vi "AuMT8852B Transmitter Test.vi"(7 "Settings":T1={"Pattern"=enum."10101010", "Hop type"=enum."Fixed", "TX/RX channel"=0, "Packet type"=enum."DH1", "Data length"=27, "Number of packets"=10}, 8 "error in (no error)":errorcluster, 11 "VISA session":refnum<visa-resource-name>) -> (0 "error out":errorcluster, 2 "error code":i32, 3 "VISA session out":refnum<visa-resource-name>)   [LabVIEW 2017]
doc: "Anritsu MT8852B Bluetooth Tester\n\nPerforms a single transmitter test control sequence. EUT must be in Test Mode before using this VI. Use Put EUT In Test Mode.vi.\n\nINPUTS\n Settings - parameters of the transmit test."
panel:
  # "Usage Notes: EUT must be in Test Mode before using this VI. Use Put EUT In Test Mode.vi."
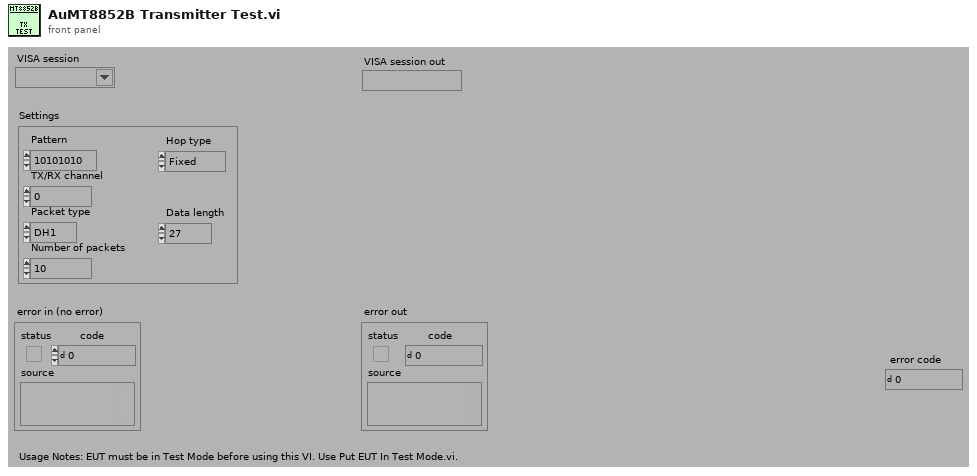
[diagram p1: front panel]
types:
  T1 = cluster{"Pattern":enum16{"10101010", "11110000", "PRBS-9"}, "Hop type":enum16{"Fixed", "Standard"}, "TX/RX channel":i32, "Packet type":enum16{"DH5", "DH3", "DH1"}, "Data length":i32, "Number of packets":i32}
  T2 = enum16{"Simulate", "Range check", "Cache", "Query instrument status"}
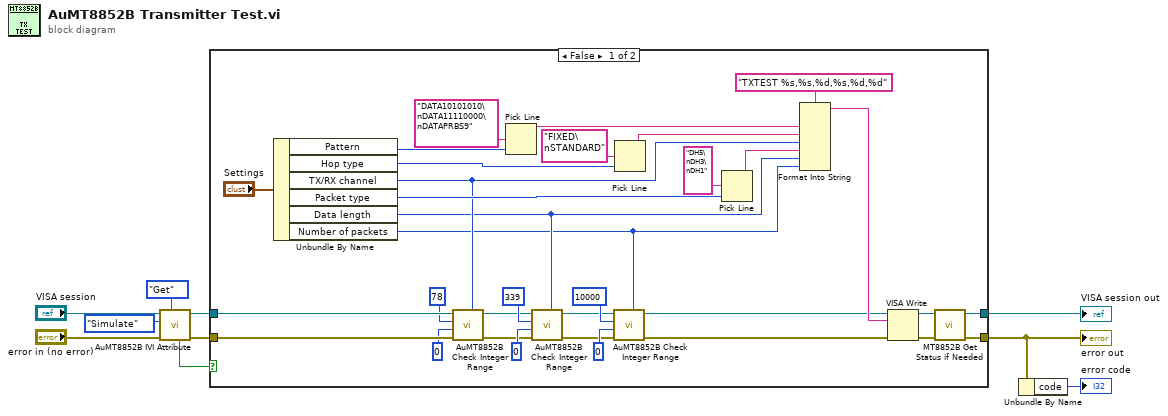
[diagram p0: block diagram]
diagram:
  n1 = call <instrlib>:"AuMT8852B IVI Attribute.vi"("Set/Get (Set)"=enum16{"Set", "Get"}."Get", "error in (no error)"="error in (no error)", "Flag (Simulate)"=T2."Simulate", "VISA session"="VISA session") -> ("error out"=w8:errorcluster, "VISA session out"=w9:refnum<visa-resource-name>, "Value out"=w3:bool)  [unwired: 5 in]
  n2 = case shown="False" w3 {
    tunnel: [w43 w45] -> w10
    tunnel: [w42 w44] -> w1
    tunnel: w8 -> [w26 w44]
    tunnel: w9 -> [w27 w45]
    frame False {
      n3 = Unbundle By Name("Settings") -> ("Pattern"=w40:enum16{"10101010", "11110000", "PRBS-9"}, "Hop type"=w37:enum16{"Fixed", "Standard"}, "TX/RX channel"=w25:i32, "Packet type"=w35:enum16{"DH5", "DH3", "DH1"}, "Data length"=w12:i32, "Number of packets"=w11:i32)
      n4 = call <instrlib>:"AuMT8852B Check Integer Range.vi"("Value (0)"=w25, "error in (no error)"=w26, "Lower limit (-1)"=0, "Upper limit (1)"=78, "VISA session"=w27) -> ("error out"=w19:errorcluster, "VISA session out"=w20:refnum<visa-resource-name>)  [unwired: 5 in]
      n5 = Pick Line(multi-line string="DATA10101010\nDATA11110000\nDATAPRBS9", line index=w40) -> (output string=w33:string)  [unwired: 1 in]
      n6 = call <instrlib>:"AuMT8852B Check Integer Range.vi"("Value (0)"=w12, "error in (no error)"=w19, "Lower limit (-1)"=0, "Upper limit (1)"=339, "VISA session"=w20) -> ("error out"=w15:errorcluster, "VISA session out"=w16:refnum<visa-resource-name>)  [unwired: 5 in]
      n7 = call <instrlib>:"AuMT8852B Check Integer Range.vi"("Value (0)"=w11, "error in (no error)"=w15, "Lower limit (-1)"=0, "Upper limit (1)"=10000, "VISA session"=w16) -> ("error out"=w13:errorcluster, "VISA session out"=w14:refnum<visa-resource-name>)  [unwired: 5 in]
      n8 = Pick Line(multi-line string="FIXED\nSTANDARD", line index=w37) -> (output string=w32:string)  [unwired: 1 in]
      n9 = Pick Line(multi-line string="DH5\nDH3\nDH1", line index=w35) -> (output string=w28:string)  [unwired: 1 in]
      n10 = Format Into String(format string="TXTEST %s,%s,%d,%s,%d,%d" ("Format String"), w33, w32, w25, w28, w12, w11) -> (resulting string=w29:string)  [unwired: 2 in, 1 out]
      n11 = VISA Write(VISA resource name=w14, write buffer=w29, error in (no error)=w13) -> (VISA resource name out=w30:refnum<visa-resource-name>, error out=w31:errorcluster)  [unwired: 1 out]
      n12 = call <instrlib>:"MT8852B Get Status if Needed.vi"("error in (no error)"=w31, "VISA session"=w30) -> ("error out"=w42:errorcluster, "VISA session out"=w43:refnum<visa-resource-name>)  [unwired: 8 in]
    }
    frame True {
    }
  }
  "error out" <- w1
  "VISA session out" <- w10
  n13 = Unbundle By Name(w1) -> ("code"=→"error code":i32)
